vi "Buffer Initialize.vi"(8 "error in (no error)":errorcluster, 9 "Number Of Elements":i32[](array[numeric]), 10 "Sector Number":i32, 11 "Circular Buffer in":refnum<class "Circular Buffer.lvclass">) -> (0 "error out":errorcluster, 3 "Circular Buffer out":refnum<class "Circular Buffer.lvclass">)   [LabVIEW 2024, in "Circular Buffer.lvclass"]
uses:
  Circular Buffer.lvclass
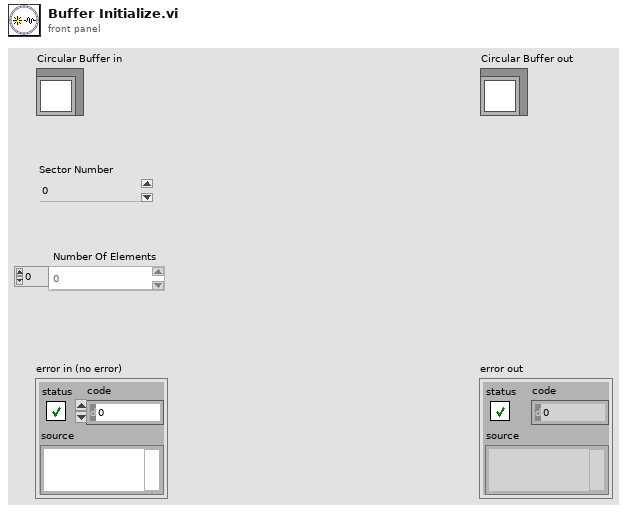
[diagram p1: front panel]
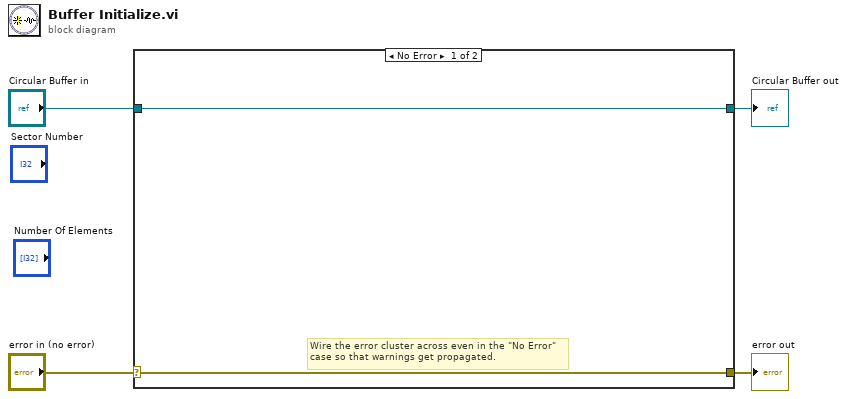
[diagram p0: block diagram]
diagram:
  n1 = case shown="No Error" "error in (no error)" {
    selector: "error in (no error)" -> [w5 w8]
    tunnel: [w5 w8] -> w3
    tunnel: [w6 w7] -> w1
    tunnel: "Circular Buffer in" -> [w6 w7]
    frame No Error {
      # "Wire the error cluster across even in the \"No Error\"\ncase so that warnings get propagated."
    }
    frame Error {
    }
  }
  "error out" <- w3
  "Circular Buffer out" <- w1
